vi "test StaticWrite (Func Global).vi"(8 "error in (no error)":errorcluster, 11 "TestCase in":refnum<class "Interface Framework Single Object.lvclass">) -> (0 "error out":errorcluster, 3 "TestCase out":refnum<class "Interface Framework Single Object.lvclass">)   [LabVIEW 2009, in "Interface Framework Single Object.lvclass"]
uses:
  Interface Framework Single Object.lvclass
  Numeric Test Object/Interface Implementations/IIntStatic (Func Global)/IIntStatic (Func Global).lvclass
  Interface Framework Single Object.lvclass/Interface Framework Single Object.ctl
  Numeric Test Object/Numeric Test Object.lvclass
  <vilib>/addons/_JKI Toolkits/VI Tester/TestCase.llb/TestCase.lvclass
  Source/Interfaceable Class/Interfaceable.lvclass
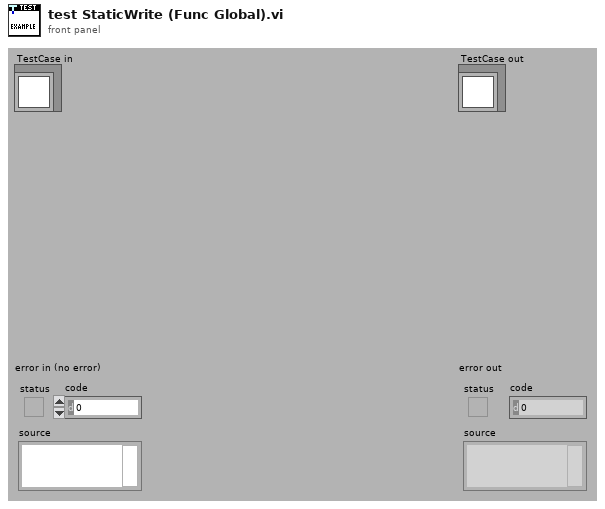
[diagram p1: front panel]
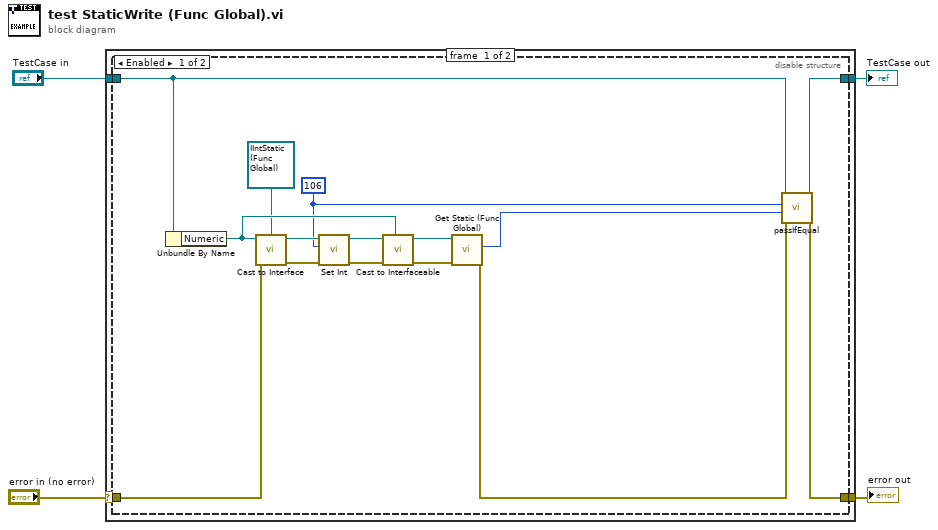
[diagram p0: block diagram]
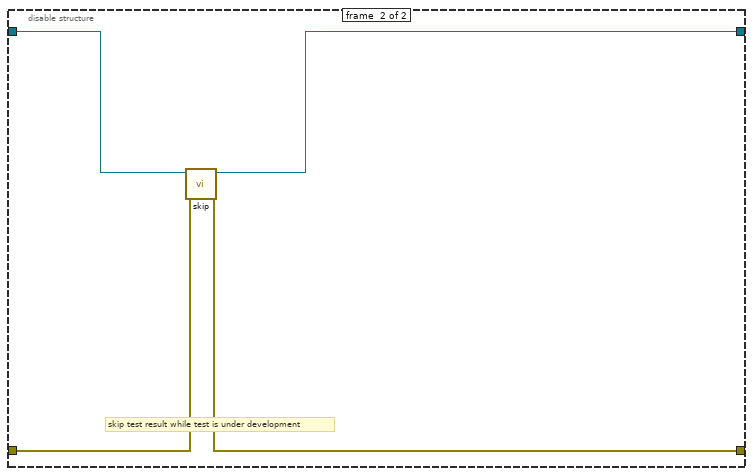
[diagram p2: hidden frame]
diagram:
  n1 = case shown="No Error" "error in (no error)" {
    selector: "error in (no error)" -> [w6 w29]
    tunnel: [w5 w29] -> w3
    tunnel: [w7 w28] -> w1
    tunnel: "TestCase in" -> [w8 w28]
    frame #0 {
      n2 = disable-structure shown="Enabled" {
        disable-tunnel: w8 -> [w21 w27]
        disable-tunnel: [w23 w24] -> w7
        disable-tunnel: w6 -> [w12 w26]
        disable-tunnel: [w22 w25] -> w5
        frame #0 {
          w15 = 106 ("Int")
          n3 = Unbundle By Name(w21) -> ("Numeric"=w18:refnum<class "Numeric Test Object.lvclass">)
          n4 = call "Cast to Interface.vi"("Target Interface"=refnum<class "IIntStatic (Func Global).lvclass"> refnum ("IIntStatic.lvclass"), "Interfaceable Object"=w18, "error in (no error)"=w12) -> ("Concrete Interface"=w20:refnum<class "IIntStatic (Func Global).lvclass">, "error out"=w11:errorcluster)  [unwired: 5 in]
          n5 = call-dynamic "Set Int.vi"("error in (no error)"=w11, "Int"=w15, "IIntStatic in"=w20) -> ("error out"=w10:errorcluster, "IIntStatic out"=w19:refnum<class "IIntStatic (Func Global).lvclass">)  [unwired: 7 in]
          n6 = call "Cast to Interfaceable.vi"("Target Object"=w18, "Interface"=w19, "error in (no error)"=w10) -> ("Interfaceable Object"=w17:refnum<class "Numeric Test Object.lvclass">, "error out"=w9:errorcluster)  [unwired: 5 in]
          n7 = call-dynamic "Get Static (Func Global).vi"("error in (no error)"=w9, "Numeric in"=w17) -> ("error out"=w16:errorcluster, "Int"=w14:i32)  [unwired: 7 in, 1 out]
          n8 = call-dynamic "passIfEqual.vi"("error in (no error)"=w16, "y"=w14, "x"=w15, "TestCase in"=w21) -> ("error out"=w22:errorcluster, "TestCase out"=w23:refnum<class "Interface Framework Single Object.lvclass">)  [unwired: 6 in]
        }
        frame #1 {
          # "skip test result while test is under development"
          n9 = call <vilib>:"skip.vi"("error in (no error)"=w26, "TestCase in"=w27) -> ("error out"=w25:errorcluster, "TestCase out"=w24:refnum<class "Interface Framework Single Object.lvclass">)  [unwired: 8 in]
        }
      }
    }
    frame #1 {
    }
  }
  "error out" <- w3
  "TestCase out" <- w1
